vi "Get drive status and trip fault code.vi"(0 "COM port":refnum<visa-resource-name>, 1 "Drive address":T5=1 items=["0", "1", "2", "3", "4", "5", "6", "7", "8", "9", "10", "11", "12", "13", "14", "15", "16", "17", "18", "19", "20", "21", "22", "23", "24", "25", "26", "27", "28", "29", "30", "31", "32", "33", "34", "35", "36", "37", "38", "39", "40", "41", "42", "43", "44", "45", "46", "47", "48", "49", "50", "51", "52", "53", "54", "55", "56", "57", "58", "59", "60", "61", "62", "63"]) -> (3 "No errors":bool, 4 "Modbus error cluster":T1={"Checksum ok"=FALSE, "Modbus exception code"=1, "Response from correct drive"=FALSE, "Comms error"={"status"=FALSE, "code"=0, "source"=""}} {"Modbus exception code" items=["None"=0, "Invalid function request"=1, "Invalid Modbus register address"=2, "Invalid / unauthorised data value"=3, "Device failure"=4, "Request accepted, wait"=5, "Drive busy"=6, "Request rejected"=7, "Memory parity error"=8, "Gateway path unavailable"=10, "Device failed to respond"=11]}, 5 "Drive status":T4, 6 "Drive fault code":T3 items=["No fault"=0, "Brake channel overcurrent"=1, "Brake resistor overload"=2, "Drive output overcurrent"=3, "Motor thermal overload"=4, "DC bus overvoltage"=6, "DC bus undervoltage"=7, "Heatsink overtemperature"=8, "Undertemperature"=9, "Factory default parameters loaded"=10, "External trip on DI 3"=11, "Serial comms loss trip"=12, "DC bus ripple too high"=13, "Input phase loss trip"=14, "Hardware overcurrent"=15, "Heatsink thermistor fault"=16, "Internal memory fault (IO)"=17, "Analog input current lost"=18, "Internal memory fault (DSP)"=19, "User default parameters loaded"=20, "Motor PTC thermistor trip"=21, "Internal cooling fan fault"=22, "Drive internal overheat"=23, "Drive output fault"=26, "Motor stator resistance varies"=40, "Motor stator resistance too large"=41, "Motor inductance too low"=42, "Motor inductance too high"=43, "Motor parameters not convergent"=44, "Modbus comms loss fault"=50, "CAN comms loss fault"=51])   [LabVIEW 2020]
doc: "Modbus RTU for Invertek drives. Paul Nathan 21-JUN-2022."
uses:
  ctls/Drive address.ctl
  ctls/Drive status bits.ctl
  ctls/Drive fault codes.ctl
  ctls/Register.ctl
  ctls/Exception codes.ctl
  ctls/Modbus error cluster.ctl
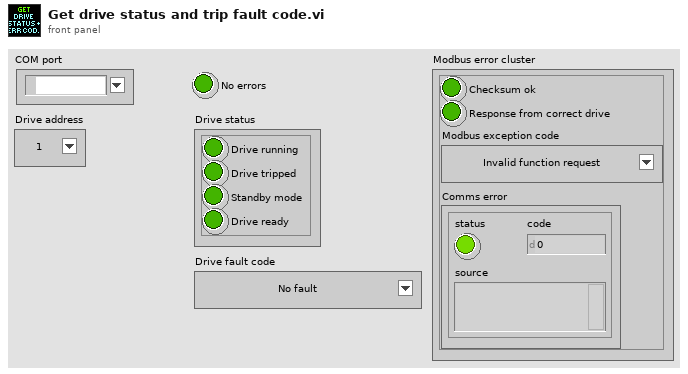
[diagram p1: front panel]
types:
  T1 = typedef "Modbus error cluster.ctl" = cluster{"Checksum ok":bool, "Modbus exception code":T2, "Response from correct drive":bool, "Comms error":errorcluster}
  T2 = typedef "Exception codes.ctl" = u8
  T3 = typedef "Drive fault codes.ctl" = u8
  T4 = typedef "Drive status bits.ctl" = cluster{"Drive running":bool, "Drive tripped":bool, "Standby mode":bool, "Drive ready":bool}
  T5 = typedef "Drive address.ctl" = u8
  T6 = typedef "Register.ctl" = u16
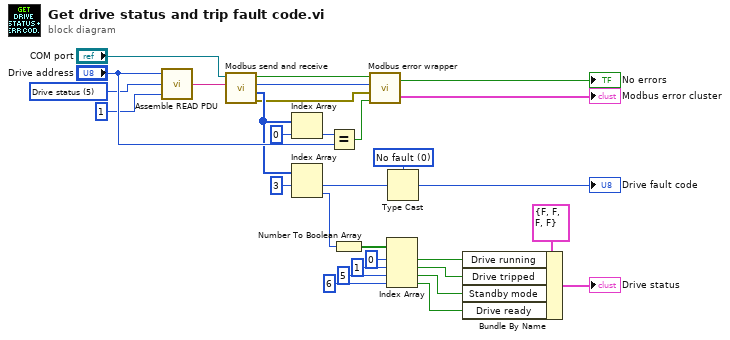
[diagram p0: block diagram]
diagram:
  w7 = T6 5 items=["Control"=0, "RPM set-point"=4, "Drive status"=5, "Output RPM"=6, "Motor current"=7, "Motor torque"=8, "Motor power"=9, "DC bus voltage"=22, "Drive power stage temperature"=23, "kWh meter"=31, "MWh meter"=32, "Running time - hours"=33, "Running time - seconds"=34, "Internal drive temperature"=38, "Motor RMS voltage"=42, "Extended drive status"=2000] ("Register")
  w10 = T3 0 items=["No fault"=0, "Brake channel overcurrent"=1, "Brake resistor overload"=2, "Drive output overcurrent"=3, "Motor thermal overload"=4, "DC bus overvoltage"=6, "DC bus undervoltage"=7, "Heatsink overtemperature"=8, "Undertemperature"=9, "Factory default parameters loaded"=10, "External trip on DI 3"=11, "Serial comms loss trip"=12, "DC bus ripple too high"=13, "Input phase loss trip"=14, "Hardware overcurrent"=15, "Heatsink thermistor fault"=16, "Internal memory fault (IO)"=17, "Analog input current lost"=18, "Internal memory fault (DSP)"=19, "User default parameters loaded"=20, "Motor PTC thermistor trip"=21, "Internal cooling fan fault"=22, "Drive internal overheat"=23, "Drive output fault"=26, "Motor stator resistance varies"=40, "Motor stator resistance too large"=41, "Motor inductance too low"=42, "Motor inductance too high"=43, "Motor parameters not convergent"=44, "Modbus comms loss fault"=50, "CAN comms loss fault"=51] ("Drive fault code")
  n1 = call "Assemble READ PDU.vi"("No. of registers"=u16 1, "Register"=w7, "Drive address"="Drive address") -> ("Ser out string"=w30:string)
  n2 = call "Modbus send and receive.vi"("Modbus telegram"=w30, "COM port"="COM port") -> ("Comms error"=w2:errorcluster, "Device response"=w24:u8[], "Modbus exception code"=w3:T2, "Checksum ok"=w4:bool)  [unwired: 2 in]
  n3 = Index Array(array=w24, index=0) -> (element=w27:u8)
  n4 = Index Array(array=w24, index #1=3 ("index")) -> (element #1=w9:u8, element #2=w22:u8)  [unwired: 1 in]
  n5 = Equal?(x=w27, y="Drive address") -> (x = y?=w1:bool)
  n6 = Number To Boolean Array(number=w22) -> (Boolean array=w21:bool[])
  n7 = call "Modbus error wrapper.vi"("Response from correct drive"=w1, "Comms error"=w2, "Modbus exception code"=w3, "Checksum ok"=w4) -> ("Modbus error cluster"=→"Modbus error cluster":T1, "No errors"=→"No errors":bool)
  n8 = Index Array(array=w21, index #1=0 ("index"), index #2=1 ("index"), index #3=5 ("index"), index #4=6 ("index")) -> (element #1=w16:bool, element #2=w15:bool, element #3=w14:bool, element #4=w13:bool)
  n9 = Type Cast(type=w10, x=w9) -> (*(type *) &x=→"Drive fault code":T3)
  n10 = Bundle By Name(cluster=T4 {"Drive running"=FALSE, "Drive tripped"=FALSE, "Standby mode"=FALSE, "Drive ready"=FALSE} ("Drive status bits"), "Drive running"=w16, "Drive tripped"=w15, "Standby mode"=w14, "Drive ready"=w13) -> (→"Drive status":T4)
